vi "myRIO__TCP_str2cmd.vi"(11 "input_string":string) -> (3 "output_packet":string)   [LabVIEW 2014]
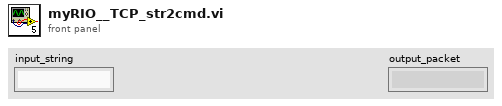
[diagram p1: front panel]
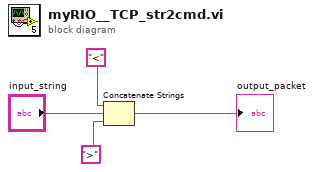
[diagram p0: block diagram]
diagram:
  n1 = Concatenate Strings("<" ("string"), "input_string", ">" ("string")) -> (→"output_packet":string)
